vi "Send Status Msg.vi"(7 "Status Msg":string, 8 "error in (no error)":errorcluster, 9 "Process Max":u16, 10 "Process Bar":u8, 11 "Session Handle in":T1) -> (0 "error out":errorcluster, 3 "Session Handle out":T1)   [LabVIEW 2018, in "Process Bar.lvclass"]
uses:
  Process Bar.lvclass
  Typedefs/Session Handle.ctl
  Process Bar.lvclass/Process Bar.ctl
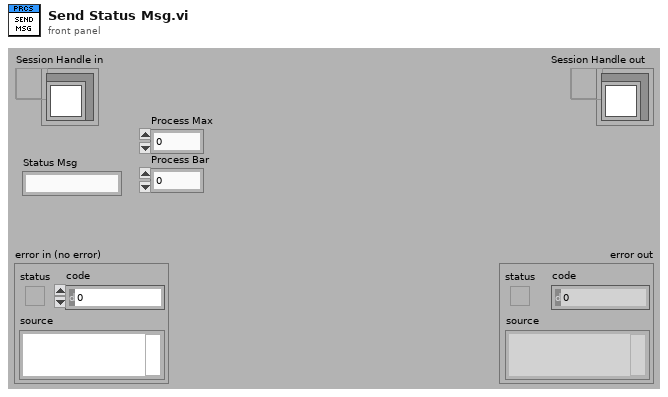
[diagram p1: front panel]
types:
  T1 = typedef "Process Bar.lvclass/Session Handle.ctl" = refnum<data-value>
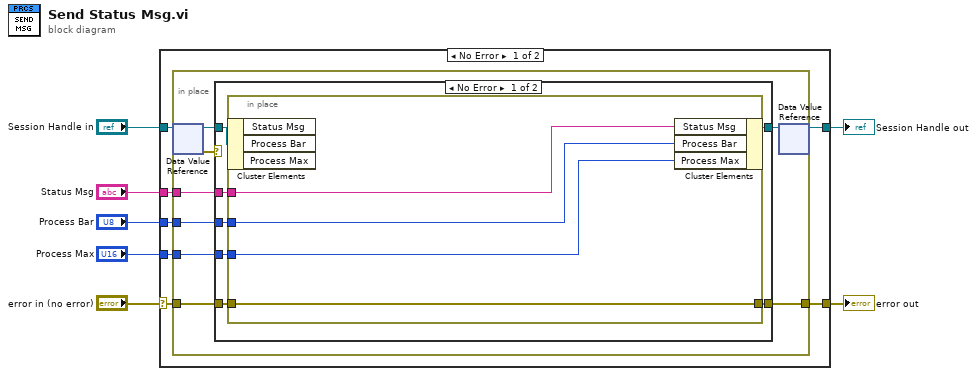
[diagram p0: block diagram]
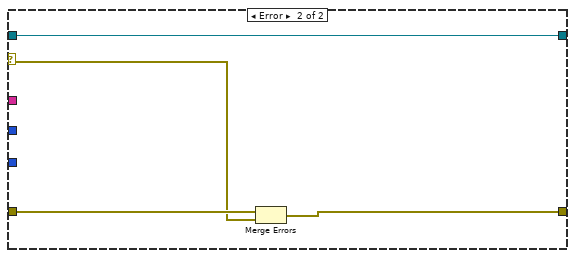
[diagram p2: hidden frame]
diagram:
  n1 = case shown="No Error" "error in (no error)" {
    selector: "error in (no error)" -> [w12 w38]
    tunnel: "Session Handle in" -> [w14 w39]
    tunnel: [w13 w39] -> w6
    tunnel: [w11 w38] -> w5
    tunnel: "Status Msg" -> [w10 _]
    tunnel: "Process Bar" -> [w9 _]
    tunnel: "Process Max" -> [w8 _]
    frame No Error {
      n2 = in-place {
        in-place-border: w12 -> [w18]
        in-place-border: [w21] -> w11
        in-place-border: w10 -> [w17]
        in-place-border: w9 -> [w16]
        in-place-border: w8 -> [w15]
        n3 = in-place-dvr #1(w14) -> (w22:refnum<class "Process Bar.lvclass">, w19:errorcluster)
        n4 = case shown="No Error" w19 {
          selector: w19 -> [_ w36]
          tunnel: w22 -> [w29 w34]
          tunnel: [w28 w35] -> w21
          tunnel: [w27 w34] -> w20
          tunnel: w18 -> [w26 w37]
          tunnel: w17 -> [w25 _]
          tunnel: w16 -> [w24 _]
          tunnel: w15 -> [w23 _]
          frame No Error {
            n5 = in-place {
              in-place-border: [w33] -> w28
              in-place-border: w26 -> [w33]
              in-place-border: w25 -> [w32]
              in-place-border: w24 -> [w31]
              in-place-border: w23 -> [w30]
              n6 = in-place-cluster #2(w29) -> ()  [unwired: 3 out]
              n7 = in-place-cluster #2("Status Msg"=w32, "Process Bar"=w31, "Process Max"=w30) -> (w27:refnum<class "Process Bar.lvclass">)
            }
          }
          frame Error {
            n8 = Merge Errors(w37, w36) -> (w35:errorcluster)
          }
        }
        n9 = in-place-dvr #1(w20) -> (w13:T1)  [unwired: 1 out]
      }
    }
    frame Error {
    }
  }
  "Session Handle out" <- w6
  "error out" <- w5
